vi "test1.vi"() -> ()   [LabVIEW 2014]
panel:
  in  "stop":bool
  out "C":dbl
  in  "B":dbl
  in  "A":dbl
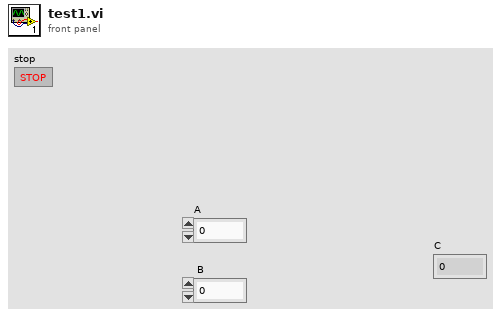
[diagram p1: front panel]
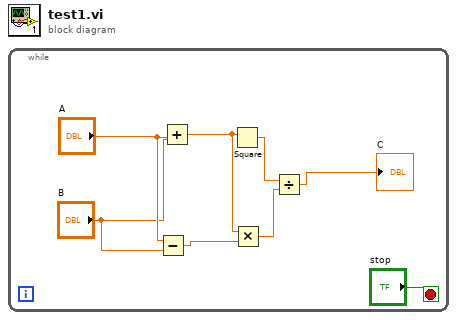
[diagram p0: block diagram]
diagram:
  n1 = while {
    stop <- "stop" stop-if-true
    n2 = Subtract(x="A", y="B") -> (x-y=w5:dbl)
    n3 = Add(x="A", y="B") -> (x+y=w6:dbl)
    n4 = Square(x=w6) -> (x^2=w3:dbl)
    n5 = Multiply(x=w6, y=w5) -> (x*y=w4:dbl)
    n6 = Divide(x=w3, y=w4) -> (x/y=→"C":dbl)
  }
